vi "Event Loop.vi"(8 "Error Q":refnum<queue>, 9 "Helper Loop Q":refnum<queue>, 10 "Actor":refnum<class "Actor.lvclass">, 11 "Helper Loop in":refnum<class "Helper Loop.lvclass">) -> ()   [LabVIEW 2021, in "Helper Loop.lvclass"]
uses:
  Helper Loop.lvclass
  <vilib>/jettl/jettl/Actor/Actor/Actor.lvclass
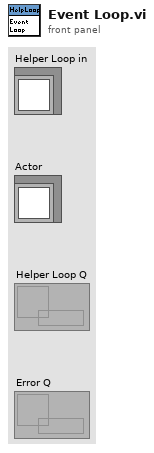
[diagram p1: front panel]
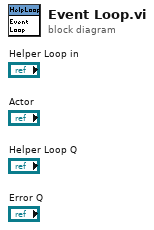
[diagram p0: block diagram]
diagram:
